vi "ROI entry-Init Cool Down ctrls.vi"(8 "error in (no error)":errorcluster) -> (0 "error out":errorcluster)   [LabVIEW 2017]
uses:
  ROI Entry screen/Globals/gl_ROI Entry UI globals.vi
  Global Variables/General Globals.vi
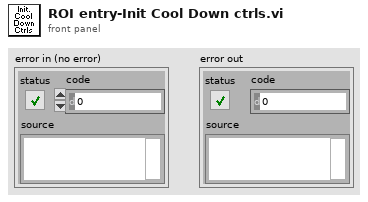
[diagram p1: front panel]
types:
  T1 = typedef "ROI entry screen ctrl refs cluster.ctl" = cluster{"Done button":refnum<vi>, "Imaging button":refnum<vi>, "Acquisition button":refnum<vi>, "POI dwell time (us)":refnum<vi>, "Scan dwell time per pixel (us)":refnum<vi>, "# of planes":refnum<vi>, "Zoom Ctrl":refnum<vi>, "Equal size":refnum<vi>, "Channel":refnum<vi>, "Image Display":refnum<vi>, "Z-Plane Selector":refnum<vi>, "Number of lines left":refnum<vi>, "Z-stack folder path":refnum<vi>, "POI Density":refnum<vi>, "Arb Plane Entry":refnum<vi>, "Whole plane":refnum<vi>, "Clear Last":refnum<vi>, "Clear All":refnum<vi>, "Trial Length (sec)":refnum<vi>, "Palette Type":refnum<vi>, "Intensity slider":refnum<vi>, "# POI":refnum<vi>, "Max Z Proj":refnum<vi>, "Zplane ind":refnum<vi>, "Wavelength (nm)":refnum<vi>, "Number of Trials":refnum<vi>, "Funct stim.trig.enable":refnum<vi>, "Funct stim.trig.delay (s)":refnum<vi>, "Line Mode":refnum<vi>, "Step size (µm)":refnum<vi>, "ROI move mode":refnum<vi>, "Cool-down time (s)":refnum<vi>, "Enable cool-down time":refnum<vi>, "Motor Z ind. (um)":refnum<vi>, "AOL Z ind. (um)":refnum<vi>, "Load Reference Image":refnum<vi>}
  T2 = enum8{"Enabled", "Disabled", "Disabled and Grayed Out"}
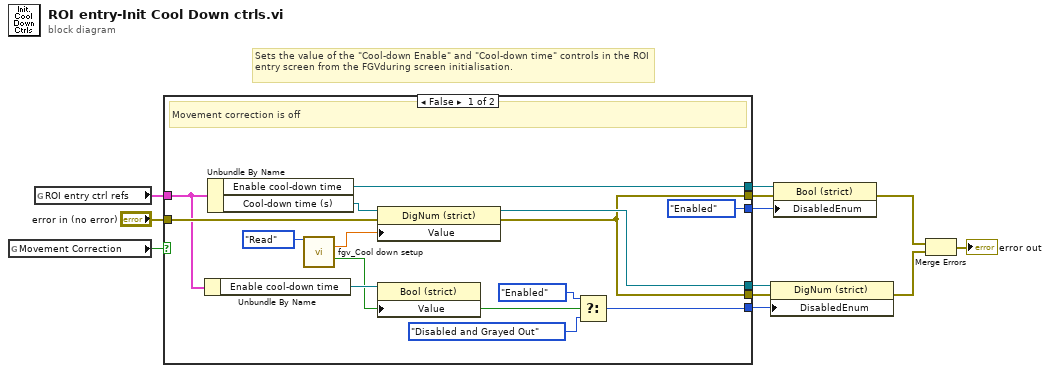
[diagram p0: block diagram]
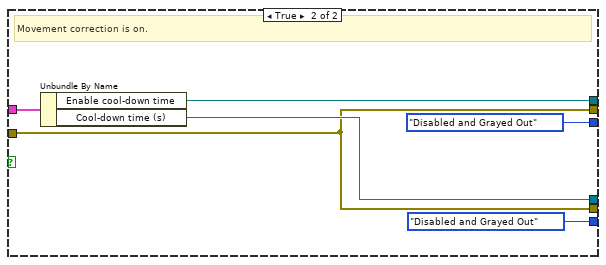
[diagram p2: hidden frame]
diagram:
  # "Sets the value of the \"Cool-down Enable\" and \"Cool-down time\" controls in the ROI entry screen from the FGVduring screen initialisation."
  n1 = global read "General Globals.vi" "Movement Correction"() -> (w7:bool)
  n2 = global read "gl_ROI Entry UI globals.vi" "ROI entry ctrl refs"() -> (w11:T1)
  n3 = case shown="False" w7 {
    tunnel: "error in (no error)" -> [w26 w27]
    tunnel: w11 -> [w24 w31]
    tunnel: [w22 T2."Disabled and Grayed Out" ("Disabled")] -> w10
    tunnel: [w13 w27] -> w9
    tunnel: [w16 w30] -> w8
    tunnel: [w15 w29] -> w6
    tunnel: [T2."Enabled" ("Disabled") T2."Disabled and Grayed Out" ("Disabled")] -> w5
    tunnel: [w13 w27] -> w4
    frame False {
      # "Movement correction is off"
      n4 = Unbundle By Name(w24) -> ("Enable cool-down time"=w25:refnum<vi>)
      n5 = Unbundle By Name(w24) -> ("Enable cool-down time"=w15:refnum<vi>, "Cool-down time (s)"=w23:refnum<vi>)
      n6 = call "fgv_Cool down setup.vi"("Function"=enum16{"Intialize", "Write", "Read", "Clear"}."Read") -> ("Cool-down time (s)"=w18:dbl, "Enable cool-down time"=w17:bool)  [unwired: 12 in, 1 out]
      n7 = property on="Property Node" class="DigNum (strict)"(reference=w23, error in=w26, "Value"=w18) -> (reference out=w16:refnum<vi>, error out=w13:errorcluster)
      n8 = property on="Property Node" class="Bool (strict)"(reference=w25, "Value"=w17) -> ()  [unwired: 1 in, 2 out]
      n9 = Select(t=T2."Enabled" ("Disabled"), s=w17, f=T2."Disabled and Grayed Out" ("Disabled")) -> (s? t:f=w22:T2)
    }
    frame True {
      # "Movement correction is on."
      n10 = Unbundle By Name(w31) -> ("Enable cool-down time"=w29:refnum<vi>, "Cool-down time (s)"=w30:refnum<vi>)
    }
  }
  n11 = property on="Property Node" class="DigNum (strict)"(reference=w8, error in=w9, "DisabledEnum"=w10) -> (error out=w3:errorcluster)  [unwired: 1 out]
  n12 = property on="Property Node" class="Bool (strict)"(reference=w6, error in=w4, "DisabledEnum"=w5) -> (error out=w2:errorcluster)  [unwired: 1 out]
  n13 = Merge Errors(w2, w3) -> (→"error out":errorcluster)
